vi "NF WF1973_74 CONT Stat.vi"(8 "error in (no error)":errorcluster caption="Error IN", 10 "Ch(Ch1)":bool, 11 "VISAsession":refnum<visa-resource-name>) -> (0 "error out":errorcluster caption="Error OUT", 2 "Query State":string, 3 "CopyVISAsession":refnum<visa-resource-name>)   [LabVIEW 2010]
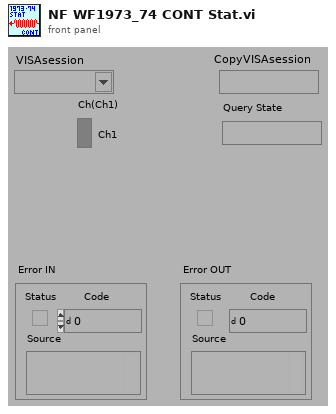
[diagram p1: front panel]
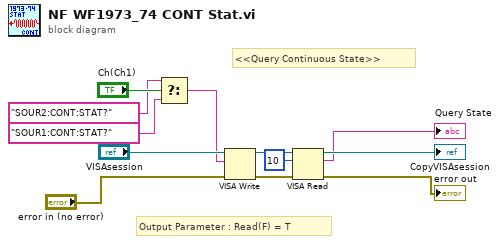
[diagram p0: block diagram]
diagram:
  # "Output Parameter : Read(F) = T"
  # "<<Query Continuous State>>"
  n1 = Select(t="SOUR2:CONT:STAT?" ("文字列"), s="Ch(Ch1)", f="SOUR1:CONT:STAT?" ("文字列")) -> (s? t:f=w1:string)
  n2 = VISA Write(VISA resource name="VISAsession", write buffer=w1, error in (no error)="error in (no error)") -> (VISA resource name out=w3:refnum<visa-resource-name>, error out=w4:errorcluster)  [unwired: 1 out]
  n3 = VISA Read(VISA resource name=w3, byte count=u32 10 ("バイトカウント（0）"), error in (no error)=w4) -> (VISA resource name out=→"CopyVISAsession":refnum<visa-resource-name>, read buffer=→"Query State":string, error out=→"error out":errorcluster)  [unwired: 1 out]
